vi "Construct Apply VIPC Step.vi"(5 "Apply VIPC Step in":refnum<class "Apply VIPC Step.lvclass">, 8 "error in (no error)":errorcluster, 11 "Path":path) -> (0 "error out":errorcluster, 3 "Apply VIPC Step":refnum<class "Apply VIPC Step.lvclass">)   [LabVIEW 2019, in "VIPM.lvlib" / "Apply VIPC Step.lvclass"]
uses:
  Apply VIPC Step.lvclass
  Apply VIPC Step.lvclass/Apply VIPC Step.ctl
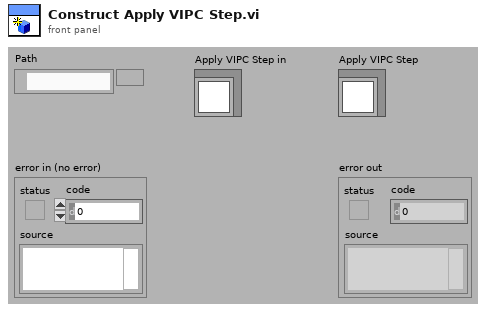
[diagram p1: front panel]
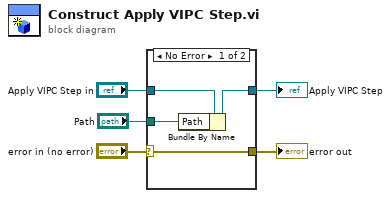
[diagram p0: block diagram]
diagram:
  n1 = case shown="No Error" "error in (no error)" {
    selector: "error in (no error)" -> [w9 w11]
    tunnel: [w9 w11] -> w4
    tunnel: [w7 w10] -> w2
    tunnel: "Apply VIPC Step in" -> [w8 w10]
    tunnel: "Path" -> [w6 _]
    frame No Error {
      n2 = Bundle By Name(cluster=w8, "Path"=w6) -> (w7:refnum<class "Apply VIPC Step.lvclass">)
    }
    frame Error {
    }
  }
  "error out" <- w4
  "Apply VIPC Step" <- w2
